vi "写入温度数据.vi"(0 "表格控件":string[][](table)) -> ()   [LabVIEW 2012]
doc: "本VI通过将表格写入Excel工作表说明利用OLE自动化VI的基本方式。"
panel:
  in  "Completion Task":u16(ring) caption="完成任务" items=["保持Excel打开", "关闭电子表格"]
  out "error out":errorcluster caption="错误输出"
  in  "error in (no error)":errorcluster caption="错误输入（无错误）"
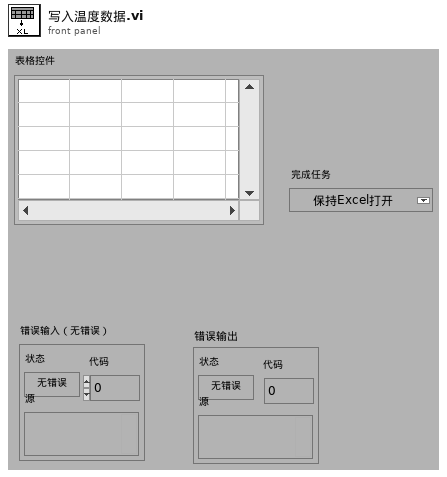
[diagram p1: front panel]
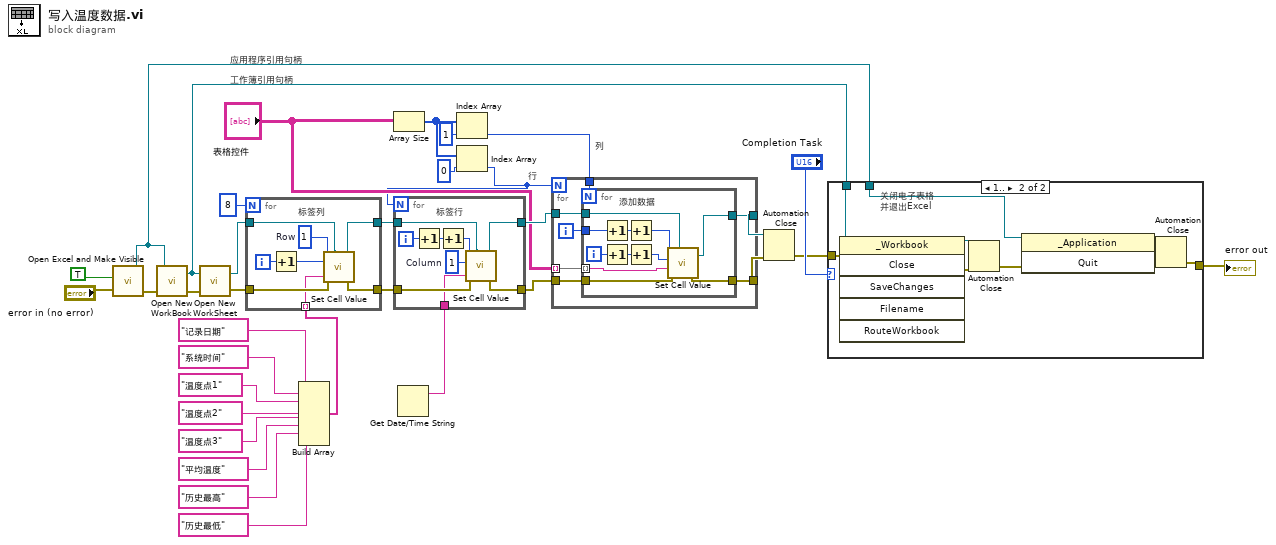
[diagram p0: block diagram]
diagram:
  # "列"
  # "行"
  # "工作簿引用句柄"
  # "应用程序引用句柄"
  n1 = call "Open Excel and Make Visible.vi"("error in (no error)"="error in (no error)", "Visible Boolean"=TRUE) -> ("error out"=w29:errorcluster, "Excel._Application"=w24:refnum<k7>)
  n2 = call "Open New  WorkBook.vi"("error in (no error)"=w29, "Excel._Application"=w24) -> ("error out"=w28:errorcluster, "Excel._Workbook"=w25:refnum<k7>)  [unwired: 1 out]
  n3 = call "Open New WorkSheet.vi"("error in (no error)"=w28, "Excel._Workbook"=w25) -> ("error out"=w19:errorcluster, "Excel._Worksheet"=w20:refnum<k7>)  [unwired: 1 out]
  n4 = Build Array("记录日期", "系统时间", "温度点1", "温度点2", "温度点3", "平均温度", "历史最高", "历史最低") -> (w15:string[])
  n5 = for {
    N: 8 -> [_]
    tunnel: w20 -> [w41]
    tunnel: w19 -> [w40]
    tunnel: [w39] -> w13
    tunnel: [w38] -> w11
    tunnel: w15 -> [w36] mode=indexing
    i -> [w42]
    w37 = 1  # Row
    # "标签列"
    n6 = Increment(x=w42) -> (x+1=w35:i32)
    n7 = call "Set Cell Value.vi"("Row"=w37, "Col"=w35, "Value"=w36, "error in (no error)"=w40, "Excel._Worksheet"=w41) -> ("Excel._Worksheet"=w38:refnum<k7>, "error out"=w39:errorcluster)
  }
  n8 = Array Size(array="表格控件") -> (size(s)=w34:i32[])
  n9 = Get Date/Time String() -> (date string=w9:string)  [unwired: 3 in, 1 out]
  n10 = Index Array(array=w34, index=1) -> (element=w27:i32)
  n11 = Index Array(array=w34, index=0) -> (element=w4:i32)
  n12 = for {
    N: w4 -> [_]
    tunnel: w11 -> [w47]
    tunnel: w13 -> [w46]
    tunnel: [w45] -> w12
    tunnel: [w44] -> w10
    tunnel: w9 -> [w43]
    i -> [w51]
    w49 = 1  # Column
    # "标签行"
    n13 = Increment(x=w51) -> (x+1=w50:i32)
    n14 = Increment(x=w50) -> (x+1=w48:i32)
    n15 = call "Set Cell Value.vi"("Row"=w48, "Col"=w49, "Value"=w43, "error in (no error)"=w46, "Excel._Worksheet"=w47) -> ("Excel._Worksheet"=w44:refnum<k7>, "error out"=w45:errorcluster)
  }
  n16 = for {
    N: w4 -> [_]
    tunnel: w10 -> [w58]
    tunnel: w12 -> [w56]
    tunnel: [w57] -> w23
    tunnel: "表格控件" -> [w55] mode=indexing
    tunnel: w27 -> [w54]
    tunnel: [w53] -> w21
    i -> [w52]
    n17 = for {
      N: w54 -> [_]
      tunnel: w58 -> [w65]
      tunnel: w56 -> [w64]
      tunnel: [w63] -> w57
      tunnel: w52 -> [w62]
      tunnel: w55 -> [w59] mode=indexing
      tunnel: [w61] -> w53
      i -> [w69]
      # "添加数据"
      n18 = Increment(x=w62) -> (x+1=w68:i32)
      n19 = Increment(x=w69) -> (x+1=w66:i32)
      n20 = Increment(x=w68) -> (x+1=w67:i32)
      n21 = Increment(x=w66) -> (x+1=w60:i32)
      n22 = call "Set Cell Value.vi"("Row"=w67, "Col"=w60, "Value"=w59, "error in (no error)"=w64, "Excel._Worksheet"=w65) -> ("Excel._Worksheet"=w61:refnum<k7>, "error out"=w63:errorcluster)
    }
  }
  n23 = Automation Close(3:w23, 5:w21) -> (0:w22:errorcluster)
  n24 = case shown="1.." "Completion Task" {
    tunnel: [w70 w71] -> w5
    tunnel: w25 -> [_ w79]
    tunnel: w24 -> [_ w75]
    tunnel: w22 -> [w70 w78]
    frame ..0 {
    }
    frame 1.. {
      # "关闭电子表格\n并退出Excel"
      n25 = invoke class="_Workbook" method="Close"(reference=w79, error in=w78) -> (reference out=w77:refnum<k7>, error out=w76:errorcluster)  [unwired: 4 in, 4 out]
      n26 = Automation Close(3:w76, 5:w77) -> (0:w74:errorcluster)
      n27 = invoke class="_Application" method="Quit"(reference=w75, error in=w74) -> (reference out=w72:refnum<k7>, error out=w73:errorcluster)  [unwired: 1 in, 1 out]
      n28 = Automation Close(3:w73, 5:w72) -> (0:w71:errorcluster)
    }
  }
  "error out" <- w5
